vi "Save Status to Log File.vi"(6 "Running?":bool=TRUE, 7 "Fully Auto?":bool=TRUE, 8 "error in":errorcluster, 9 "Info":T1, 10 "System Status":string, 11 "Log File In":path) -> (0 "error out":errorcluster, 3 "Log File Out":path)   [LabVIEW 2016]
uses:
  Controls/Info.ctl
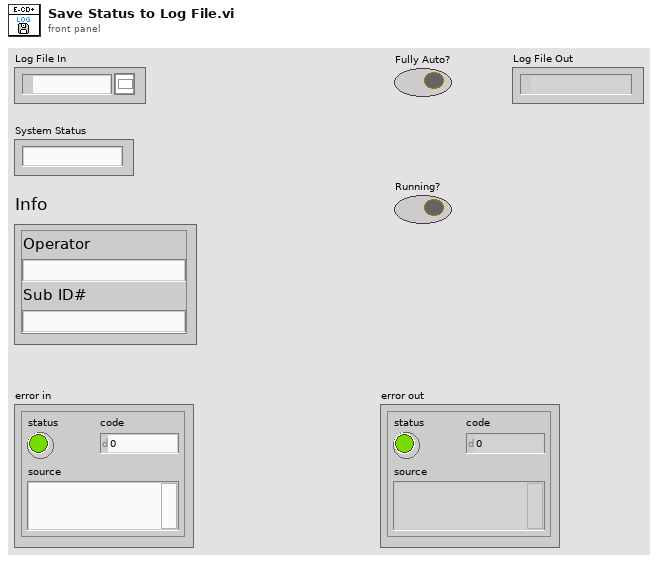
[diagram p1: front panel]
types:
  T1 = typedef "Info.ctl" = cluster{"Operator":string, "Sub ID#":string}
  T2 = enum16{"open", "replace", "create", "open or create", "replace or create", "replace or create with confirmation"}
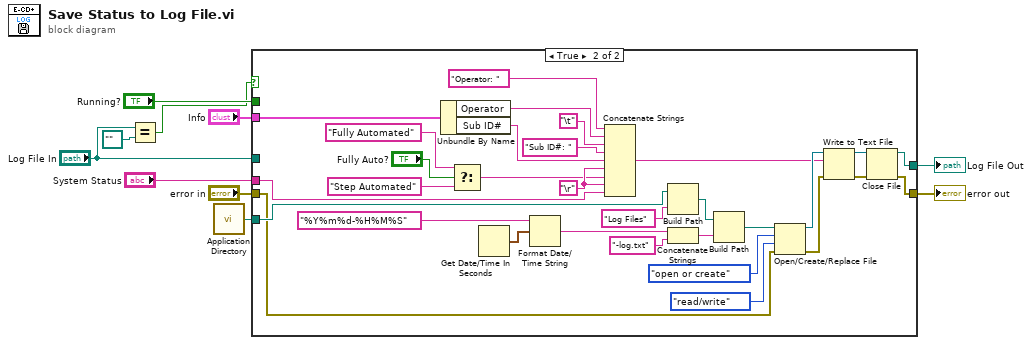
[diagram p0: block diagram]
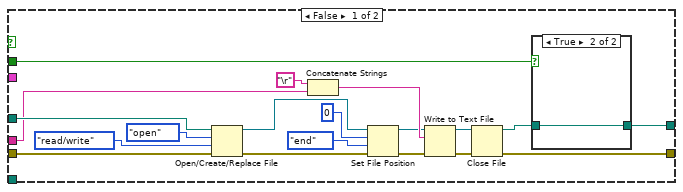
[diagram p2: hidden frame]
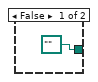
[diagram p3: hidden frame]
diagram:
  n1 = Equal?(x="Log File In", y=path "") -> (x = y?=w1:bool)
  n2 = call <vilib>:"Application Directory.vi"() -> ("Application Directory"=w3:path)
  n3 = case shown="True" w1 {
    tunnel: "error in" -> [w17 w38]
    tunnel: [w16 w41] -> w8
    tunnel: "Log File In" -> [w15 _]
    tunnel: w3 -> [_ w42]
    tunnel: [w11 w40] -> w4
    tunnel: "System Status" -> [w14 w36]
    tunnel: "Info" -> [_ w39]
    tunnel: "Running?" -> [w13 _]
    frame False {
      n4 = Open/Create/Replace File(file path (use dialog)=w15, error in=w17, operation (0:open)=T2."open", access (0:read/write)=enum16{"read/write", "read-only", "write-only"}."read/write") -> (refnum out=w22:refnum<file>, error out=w24:errorcluster)  [unwired: 2 in, 1 out]
      n5 = Concatenate Strings("\r", w14) -> (w29:string)
      n6 = Set File Position(offset (in bytes) (0)=i64 0, refnum=w22, from (0:start)=enum16{"start", "end", "current"}."end", error in=w24) -> (refnum out=w23:refnum<file>, error out=w25:errorcluster)
      n7 = Write to Text File(file (use dialog)=w23, text=w29, error in=w25) -> (refnum out=w18:refnum<file>, error out=w19:errorcluster)  [unwired: 1 in, 1 out]
      n8 = Close File(refnum=w18, error in=w19) -> (path=w12:path, error out=w16:errorcluster)
      n9 = case shown="True" w13 {
        tunnel: w12 -> [_ w31]
        tunnel: [path "" ("path") w31] -> w11
        frame False {
        }
        frame True {
        }
      }
    }
    frame True {
      w35 = "\r"
      n10 = Unbundle By Name(w39) -> ("Operator"=w61:string, "Sub ID#"=w62:string)
      n11 = Select(t="Fully Automated" ("string"), s="Fully Auto?", f="Step Automated" ("string")) -> (s? t:f=w32:string)
      n12 = Get Date/Time In Seconds() -> (seconds since 1Jan1904=w59:timestamp)
      n13 = Format Date/Time String(time format string (%c)="%Y%m%d-%H%M%S", seconds (now)=w59) -> (date/time string=w56:string)  [unwired: 1 out]
      n14 = Concatenate Strings("Operator: " ("string"), w61, "\t", "Sub ID#: " ("string"), w62, w35, w32, w35, w36) -> (w44:string)
      n15 = Build Path(base path=w42, name or relative path="Log Files") -> (appended path=w57:path)
      n16 = Concatenate Strings(w56, "-log.txt" ("string")) -> (w54:string)
      n17 = Build Path(base path=w57, name or relative path=w54) -> (appended path=w43:path)
      n18 = Open/Create/Replace File(file path (use dialog)=w43, error in=w38, operation (0:open)=T2."open or create", access (0:read/write)=enum16{"read/write", "read-only", "write-only"}."read/write") -> (refnum out=w50:refnum<file>, error out=w51:errorcluster)  [unwired: 2 in, 1 out]
      n19 = Write to Text File(file (use dialog)=w50, text=w44, error in=w51) -> (refnum out=w48:refnum<file>, error out=w49:errorcluster)  [unwired: 1 in, 1 out]
      n20 = Close File(refnum=w48, error in=w49) -> (path=w40:path, error out=w41:errorcluster)
    }
  }
  "error out" <- w8
  "Log File Out" <- w4
